vi "Set Data Binding.vi"(7 "DataTable Source":refnum<class "DataTable.lvclass">, 8 "error in (no error)":errorcluster, 11 "DataGridView in":refnum<class "DataGridView.lvclass">) -> (0 "error out":errorcluster, 3 "DataGridView out":refnum<class "DataGridView.lvclass">)   [LabVIEW 2013, in "DataGrid.lvlib" / "DataGridView.lvclass"]
doc: "This is a simple data binding step that connects the dataTable with all the data in it, into the DataGridView for display. The columns get bound and autogenerated by the datagridview for any object types with native support in this step. The next step is to set any custom column types to define specific object types."
uses:
  DataGridView.lvclass
  DataTable/DataTable.lvclass
  DataTable/DataTable.lvclass/DataTable.ctl
  System.Windows.Forms
  DataGridView.lvclass/DataGridView.ctl
  DataTable/Read DataTable.vi
  Properties/Read DataGridView.vi
  System.Data
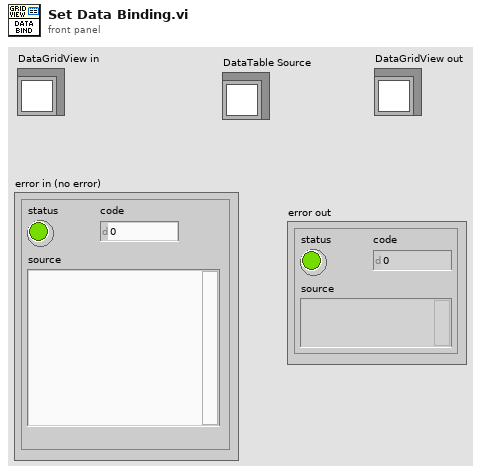
[diagram p1: front panel]
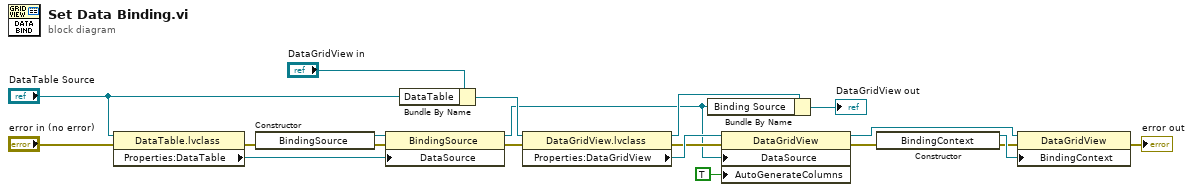
[diagram p0: block diagram]
diagram:
  n1 = property class="DataTable.lvclass"(reference="DataTable Source", error in="error in (no error)") -> (error out=w5:errorcluster, "Properties:DataTable"=w2:refnum<k24>)  [unwired: 1 out]
  n2 = constructor class="BindingSource"(error in=w5) -> (reference out=w6:refnum<k24>, error out=w4:errorcluster)  [unwired: 2 in, 1 out]
  n3 = property class="BindingSource"(reference=w6, error in=w4, "DataSource"=w2) -> (reference out=w1:refnum<k24>, error out=w3:errorcluster)
  n4 = Bundle By Name(cluster="DataGridView in", "DataTable"="DataTable Source") -> (w10:refnum<class "DataGridView.lvclass">)
  n5 = property class="DataGridView.lvclass"(reference=w10, error in=w3) -> (reference out=w8:refnum<class "DataGridView.lvclass">, error out=w14:errorcluster, "Properties:DataGridView"=w15:refnum<k24>)
  n6 = Bundle By Name(cluster=w8, "Binding Source"=w1) -> (→"DataGridView out":refnum<class "DataGridView.lvclass">)
  n7 = property class="DataGridView"(reference=w15, error in=w14, "DataSource"=w1, "AutoGenerateColumns"=TRUE) -> (reference out=w18:refnum<k24>, error out=w20:errorcluster)
  n8 = constructor class="BindingContext"(error in=w20) -> (reference out=w17:refnum<k24>, error out=w16:errorcluster)  [unwired: 2 in, 1 out]
  n9 = property class="DataGridView"(reference=w18, error in=w16, "BindingContext"=w17) -> (error out=→"error out":errorcluster)  [unwired: 1 out]
